vi "Abort Stream.vi"(0 "Register Bus":T2, 1 "scope":string(combo)="rx", 9 "timeout (s)":dbl=10.0, 11 "error in":errorcluster) -> (4 "Register Bus (out)":T2, 15 "error out":errorcluster)   [LabVIEW 2017]
doc: "Abort the acquisition/generation, wait for the stream to go idle, then check the stream status.\n\n<B>Input Parameters</B>\n\n<B>Register Bus</B> The Register Bus object created by the ni579x Open VI and used as the session handle for the NI-579x Configuration Design Library.\n\n<B>scope</B> is the channel to abort the stream for. The options are \"rx\" and \"tx\".\n\n<B>timeout (s)</B> is how long to wait for (in seconds).\n\n<B>error in</B> describes error conditions that occur before this node runs. This input provides standard 'error in' functionality.\n\n<B>Output Parameters</B>\n\n<B>Register Bus (out)</B> The Register Bus object created by the ni579x Open VI and used as the session handle for the NI-579x Configuration Design Library.\n\n<B>error out</B> contains error information. This output provides standard 'error out' functionality."
uses:
  <instrlib>/_niInstr/Register Bus/v0/Host/Public/Register Bus Session.ctl
  <instrlib>/_niInstr/Register Bus/v0/Host/Private/Session Data.ctl
  FPGA/SubVIs/Stream Control State.ctl
  Tx FPGA VI Reference.ctl
  Rx FPGA VI Reference.ctl
  <vilib>/rvi/errors/niLvFpgaAdjustHostInterfaceError.vi
  <vilib>/rvi/interface/nirviReadWriteControl/nirviReadWriteControl.xnode
  <vilib>/rvi/interface/Simulation/niFpgaSimulationCallBeginRW.vi
  NiFpgaLv.dll
  <instrlib>/_niInstr/Register Bus/v0/Host/niInstr Register Bus v0 Host.lvlib
panel:
  out "samples processed":u32
  out "state":T1
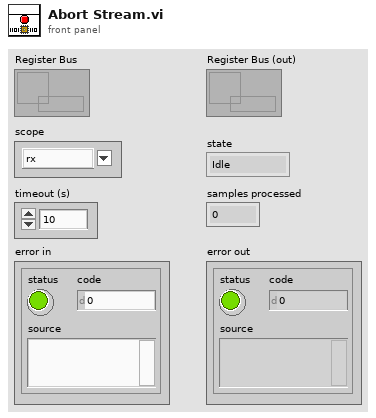
[diagram p1: front panel]
types:
  T1 = typedef "Stream Control State.ctl" = enum16{"Idle", "Active"}
  T2 = typedef "niInstr Register Bus v0 Host.lvlib/Register Bus Session.ctl" = refnum<queue>
  T3 = typedef "Tx FPGA VI Reference.ctl" = refnum<k20>
  T4 = typedef "Rx FPGA VI Reference.ctl" = refnum<k20>
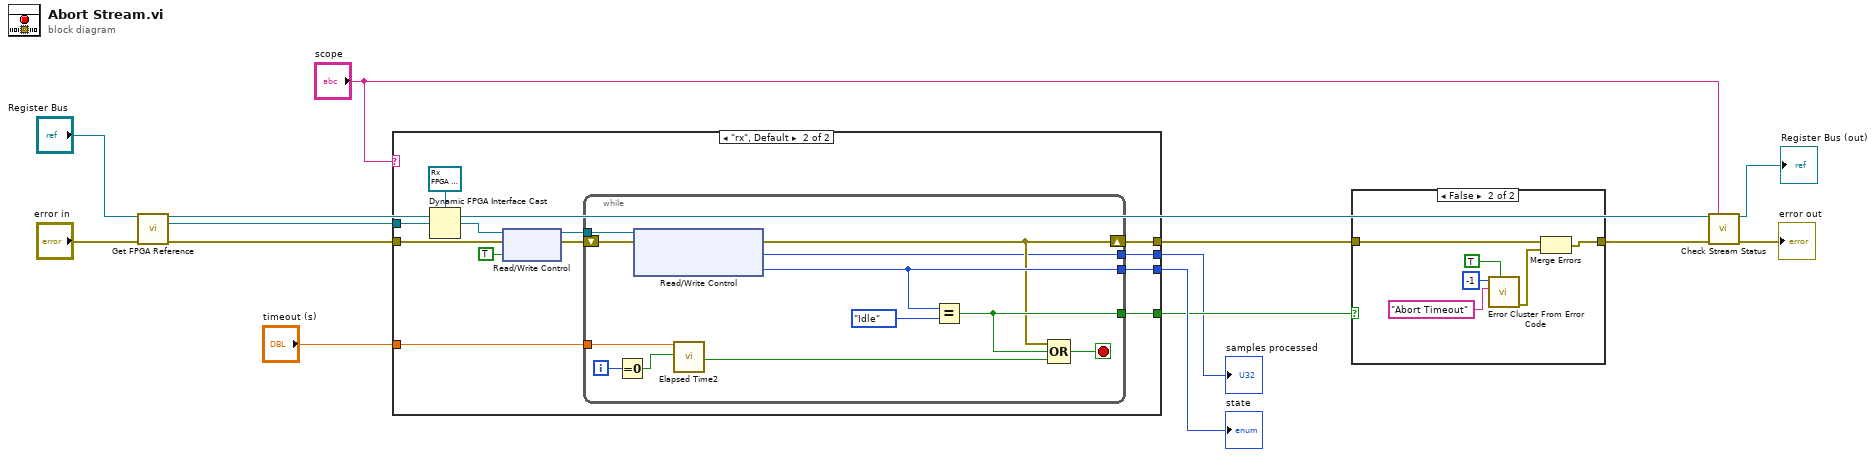
[diagram p0: block diagram]
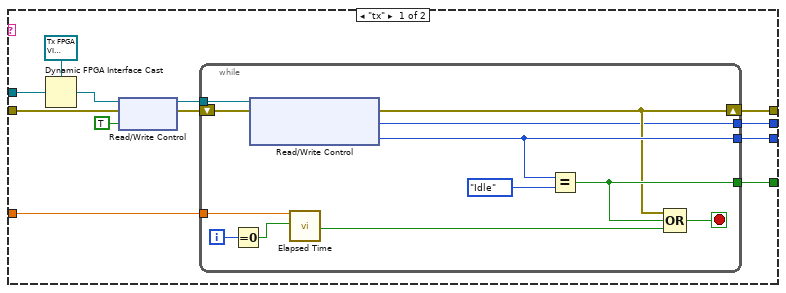
[diagram p2: hidden frame]
diagram:
  n1 = call <instrlib>:"Get FPGA Reference.vi"("session in"="Register Bus", "error in"="error in") -> ("session out"=w3:T2, "fpga ref"=w13:refnum<k20>, "error out"=w12:errorcluster)  [unwired: 11 in]
  n2 = case shown="\"rx\", Default" "scope" {
    tunnel: w13 -> [w26 w50]
    tunnel: w12 -> [w24 w48]
    tunnel: [w22 w46] -> w11
    tunnel: [w19 w43] -> w10
    tunnel: [w17 w42] -> w9
    tunnel: "timeout (s)" -> [w16 w41]
    tunnel: [w15 w40] -> w6
    frame "tx" {
      n3 = Dynamic FPGA Interface Cast(Session In=T3 refnum ("Type"), Type=w26) -> (Session Out=w25:T3)
      n4 = xnode "Read/Write Control"("FPGA VI Reference In"=w25, "error in"=w24, "tx.abort"=TRUE ("Tx.Reset")) -> ("FPGA VI Reference Out"=w21:T3, "error out"=w20:errorcluster)
      n5 = while {
        tunnel: w21 -> [w38]
        tunnel: [w33] -> w17
        shift-right: [w29] -> w22
        shift-left: w20 -> [w37]
        tunnel: [w30] -> w19
        tunnel: w16 -> [w28]
        tunnel: [w27] -> w15
        i -> [w35]
        stop <- w34 stop-if-true
        n6 = Equal To 0?(x=w35) -> (x = 0?=w36:bool)
        n7 = xnode "Read/Write Control"("FPGA VI Reference In"=w38, "error in"=w37) -> ("error out"=w29:errorcluster, "tx.samples processed"=w27:u32, "tx.state"=w30:enum16{"Idle", "Active"})  [unwired: 1 out]
        n8 = call "Elapsed Time"("Time Target (s)"=w28, "Reset"=w36) -> ("Time has Elapsed"=w31:bool)  [unwired: 10 in, 7 out]
        n9 = Equal?(x=w30, y=Stream_Control_State."Idle" ("state")) -> (x = y?=w33:bool)
        n10 = Compound Arithmetic op=OR(w29, w33, w31) -> (w34:bool)
      }
    }
    frame "rx", Default {
      n11 = Dynamic FPGA Interface Cast(Session In=T4 refnum ("Type"), Type=w50) -> (Session Out=w49:T4)
      n12 = xnode "Read/Write Control"("FPGA VI Reference In"=w49, "error in"=w48, "rx.abort"=TRUE ("Tx.Reset")) -> ("FPGA VI Reference Out"=w45:T4, "error out"=w44:errorcluster)
      n13 = while {
        tunnel: w45 -> [w62]
        tunnel: [w57] -> w42
        shift-right: [w53] -> w46
        shift-left: w44 -> [w61]
        tunnel: [w54] -> w43
        tunnel: w41 -> [w52]
        tunnel: [w51] -> w40
        i -> [w59]
        stop <- w58 stop-if-true
        n14 = Equal To 0?(x=w59) -> (x = 0?=w60:bool)
        n15 = xnode "Read/Write Control"("FPGA VI Reference In"=w62, "error in"=w61) -> ("error out"=w53:errorcluster, "rx.samples processed"=w51:u32, "rx.state"=w54:enum16{"Idle", "Active"})  [unwired: 1 out]
        n16 = call "Elapsed Time2"("Time Target (s)"=w52, "Reset"=w60) -> ("Time has Elapsed"=w55:bool)  [unwired: 10 in, 7 out]
        n17 = Equal?(x=w54, y=Stream_Control_State."Idle" ("state")) -> (x = y?=w57:bool)
        n18 = Compound Arithmetic op=OR(w53, w57, w55) -> (w58:bool)
      }
    }
  }
  "state" <- w10
  "samples processed" <- w6
  n19 = case shown="False" w9 {
    tunnel: w11 -> [w63 w68]
    tunnel: [w63 w66] -> w5
    frame True {
    }
    frame False {
      n20 = call <vilib>:"Error Cluster From Error Code.vi"("show call chain? (False)"=TRUE, "error message (\"\")"="Abort Timeout" ("error message (\"\")"), "error code (0)"=-1) -> ("error out"=w67:errorcluster)  [unwired: 6 in]
      n21 = Merge Errors(w68, w67) -> (w66:errorcluster)
    }
  }
  n22 = call "Check Stream Status.vi"("Register Bus"=w3, "scope"="scope", "error in"=w5) -> ("Register Bus (out)"=→"Register Bus (out)":T2, "error out"=→"error out":errorcluster)  [unwired: 11 in]
